vi "Trayectoria.vi"() -> ()   [LabVIEW 2018]
uses:
  <vilib>/Analysis/Matrix/Numeric/Conversions/Array To Matrix - RA2.vi
  <vilib>/Analysis/baseanly.llb/Real Inverse Matrix.vi
  <vilib>/Analysis/Matrix/Numeric/Multiply/Multiply - RM,RM.vi
  <vilib>/Analysis/NI_AALBase.lvlib
  <vilib>/Analysis/Matrix/NI_Matrix.lvlib
panel:
  out "XY Graph":cluster{dbl[], dbl[]}(graph)
  out "Vector Spline":dbl[](array[numeric])
  out "Vector tiempo":dbl[](array[numeric])
  out "Constantes":dbl[](array[numeric])
  in  "tetha_f_p":dbl
  in  "tetha_o_p":dbl
  in  "tetha_o_pp":dbl
  in  "tetha_f_pp":dbl
  in  "tf":dbl
  in  "tetha_f":dbl
  in  "tetha_o":dbl
  in  "stop":bool
  # "ÁNGULO"
  # "VELOCIDAD"
  # "ACELERACIÓN"
  # "a0"
  # "a1"
  # "a2"
  # "a3"
  # "a4"
  # "a5"
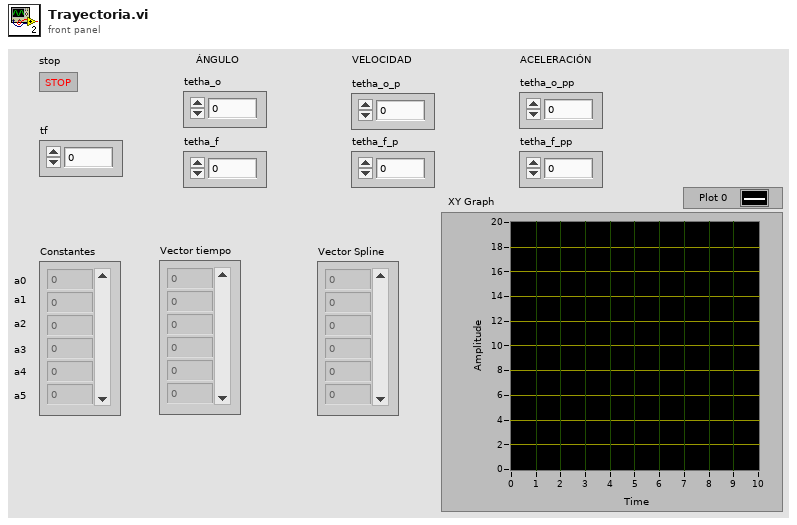
[diagram p1: front panel]
types:
  T1 = typedef "NI_Matrix.lvlib/RealMatrix.ctl" = dbl[][]
  T2 = cluster{"[0]":dbl, "[1]":dbl, "[2]":dbl, "[3]":dbl, "[4]":dbl, "[5]":dbl, "[6]":dbl, "[7]":dbl, "[8]":dbl}
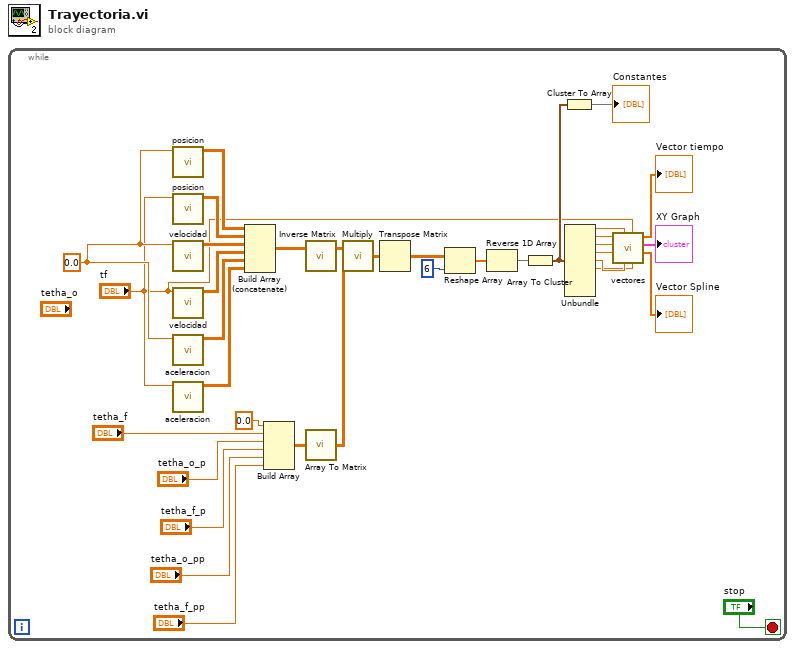
[diagram p0: block diagram]
diagram:
  n1 = while {
    stop <- "stop" stop-if-true
    w6 = 0.0
    n2 = call "posicion.vi"("a0"=w6) -> ("Real Matrix"=w24:T1)  [unwired: 10 in]
    n3 = call "posicion.vi"("a0"="tf") -> ("Real Matrix"=w4:T1)  [unwired: 10 in]
    n4 = call "velocidad.vi"("a0"=w6) -> ("Real Matrix"=w23:T1)  [unwired: 10 in]
    n5 = call "velocidad.vi"("a0"="tf") -> ("Real Matrix"=w3:T1)  [unwired: 10 in]
    n6 = call "aceleracion.vi"("a0"=w6) -> ("Real Matrix"=w22:T1)  [unwired: 10 in]
    n7 = call "aceleracion.vi"("a0"="tf") -> ("Real Matrix"=w1:T1)  [unwired: 10 in]
    n8 = Build Array (concatenate) ("Build Matrix")(w24, w4, w23, w3, w22, w1) -> (w9:T1)
    n9 = Build Array(0.0, "tetha_f", "tetha_o_p", "tetha_f_p", "tetha_o_pp", "tetha_f_pp") -> (w20:T1)
    n10 = call-poly <vilib>:"Inverse Matrix.vi"("Input Matrix"=w9) -> ("Inverse Matrix"=w10:T1)  [unwired: 1 in, 1 out]
    n11 = call-poly <vilib>:"Array To Matrix.vi"("Real 2D Array"=w20) -> ("Real Matrix"=w19:T1)
    n12 = call-poly <vilib>:"Multiply.vi"("Real Matrix B"=w19, "Real Matrix A"=w10) -> ("A * B"=w12:T1)
    n13 = Transpose Matrix(1:w12) -> (0:w11:T1)
    n14 = Reshape Array(w11, 6 ("dimension size")) -> (w8:dbl[])
    n15 = Reverse 1D Array(array=w8) -> (reversed array=w7:dbl[])
    n16 = Array To Cluster(array=w7) -> (cluster=w17:T2)
    n17 = Cluster To Array(cluster=w17) -> (array=→"Constantes":dbl[])
    n18 = Unbundle(w17) -> ("[0]"=w33:dbl, "[1]"=w32:dbl, "[2]"=w31:dbl, "[3]"=w30:dbl, "[4]"=w29:dbl, "[5]"=w28:dbl)  [unwired: 3 out]
    n19 = call "vectores.vi"("a5"=w28, "tf"="tf", "a4"=w29, "tetha_o"=w33, "a3"=w30, "a2"=w31, "tetha_o_p"=w32) -> ("Vector Spline"=→"Vector Spline":dbl[], "Cluster"=→"XY Graph":cluster{dbl[], dbl[]}, "Vector tiempo"=→"Vector tiempo":dbl[])  [unwired: 2 in]
  }
